vi "ReBuild Menu.vi"(8 "error in (no error)":errorcluster, 11 "menu reference":refnum<k9>) -> (0 "error out":errorcluster, 3 "Station Config":T1)   [LabVIEW 2025, in "Full User Interface.lvlib"]
uses:
  Full User Interface.lvlib
  Station Config.ctl
  Station Info.ctl
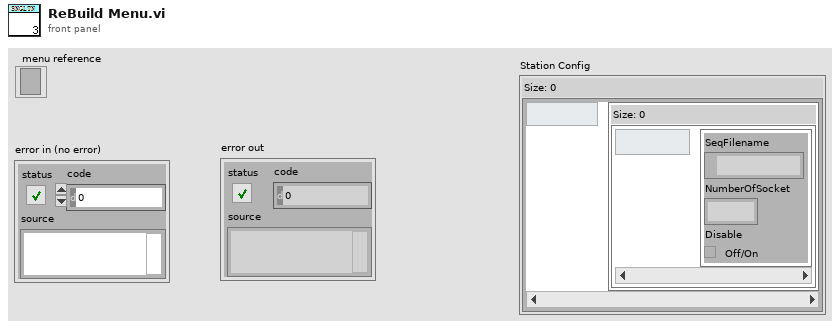
[diagram p1: front panel]
types:
  T1 = typedef "Full User Interface.lvlib/Station Config.ctl" = map{string, map{i32, T2}}
  T2 = typedef "Full User Interface.lvlib/Station Info.ctl" = cluster{"SeqFilename":path, "NumberOfSocket":i32, "Disable":bool}
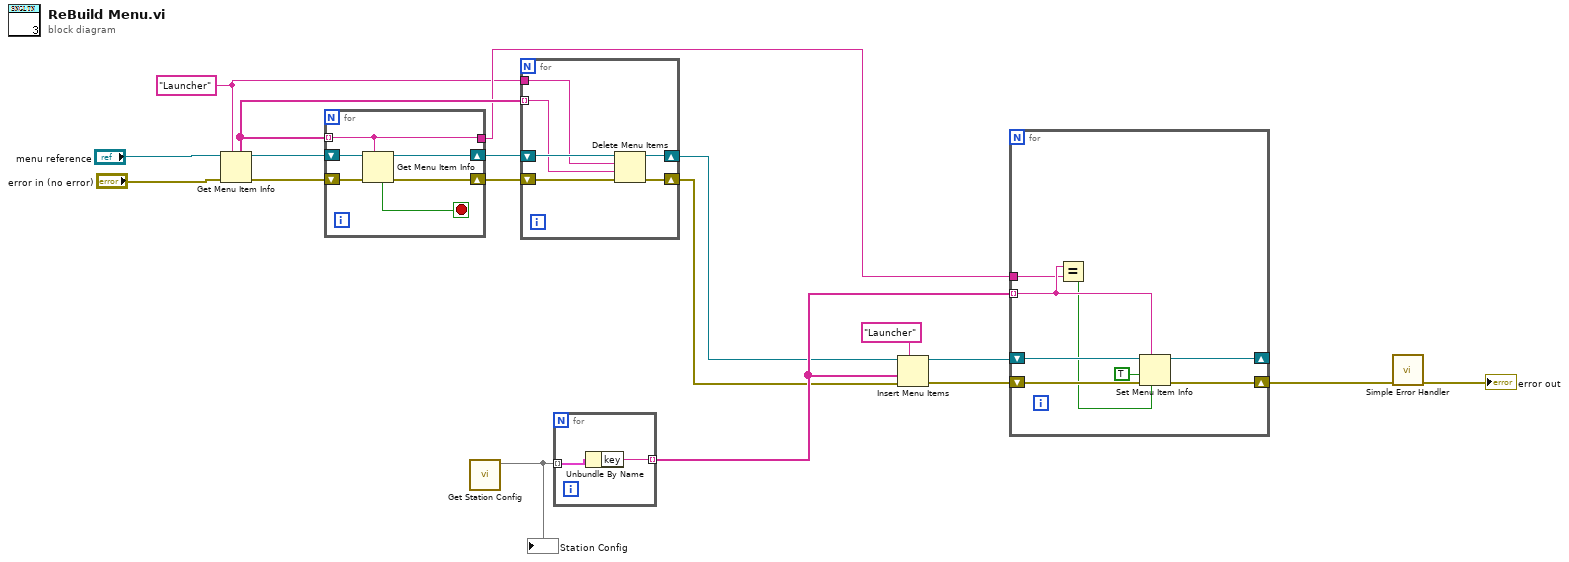
[diagram p0: block diagram]
diagram:
  w1 = "Launcher"
  n1 = Get Menu Item Info(7:w1, 8:"error in (no error)", 11:"menu reference") -> (0:w6:errorcluster, 3:w9:refnum<k9>, 5:w7:string[])  [unwired: 4 out]
  n2 = for {
    tunnel: w7 -> [w22] mode=indexing
    tunnel: [w22] -> w2
    shift-right: [w21] -> w8
    shift-left: w9 -> [w24]
    shift-right: [w19] -> w5
    shift-left: w6 -> [w20]
    stop <- w23 stop-if-true
    n3 = Get Menu Item Info(7:w22, 8:w20, 11:w24) -> (0:w19:errorcluster, 3:w21:refnum<k9>, 4:w23:bool)  [unwired: 4 out]
  }
  n4 = call "Get Station Config.vi"() -> ("Station Config"=w16:T1)  [unwired: 10 in, 1 out]
  "Station Config" <- w16
  n5 = for {
    tunnel: w7 -> [w26] mode=indexing
    shift-right: [w28] -> w3
    shift-left: w5 -> [w29]
    shift-right: [w27] -> w4
    shift-left: w8 -> [w30]
    tunnel: w1 -> [w25]
    n6 = Delete Menu Items(6:w29, 7:w26, 8:w25, 9:w30) -> (0:w28:errorcluster, 3:w27:refnum<k9>)
  }
  n7 = for {
    tunnel: w16 -> [w32] mode=indexing
    tunnel: [w31] -> w12 mode=indexing
    n8 = Unbundle By Name(w32) -> ("key"=w31:string)
  }
  n9 = Insert Menu Items(5:"Launcher", 6:w3, 7:w12, 9:w4) -> (0:w15:errorcluster, 3:w13:refnum<k9>)  [unwired: 2 in, 1 out]
  n10 = for {
    shift-right: [w39] -> _
    shift-left: w13 -> [w40]
    shift-right: [w37] -> w14
    shift-left: w15 -> [w38]
    tunnel: w12 -> [w35] mode=indexing
    tunnel: w2 -> [w34]
    n11 = Equal?(x=w35, y=w34) -> (x = y?=w33:bool)
    n12 = Set Menu Item Info(6:w33, 7:w35, 8:w38, 9:TRUE ("enabled"), 11:w40) -> (0:w37:errorcluster, 3:w39:refnum<k9>)  [unwired: 2 in]
  }
  n13 = call <vilib>:"Simple Error Handler.vi"("error in (no error)"=w14) -> ("error out"=→"error out":errorcluster)  [unwired: 4 in, 4 out]
